vi "Generate View Regular Functions.vi"(8 "Error in":errorcluster, 9 "Table Name":string, 10 "Folder to Saved File":path, 11 "Connection in":refnum<class "Connection.lvclass">) -> (0 "Error out":errorcluster, 2 "SQL-LV File Paths":T1, 3 "Connection out":refnum<class "Connection.lvclass">)   [LabVIEW 2021]
uses:
  <vilib>/drjdpowell/SQLite Library/SQL Connection/Connection.lvclass
  SQL-LV View File Paths.ctl
  SQL-LV View Control Paths.ctl
  SQL-LV View VI Paths.ctl
  edt.lib/sqlite.lib/SQLite Field Info.ctl
  edt.lib/sqlite.lib/SQLite Data Type.ctl
  SQL-LV Table Control Paths.ctl
  Field Info to Cluster Item Info (Array).vi
  edt.lib/vie.lib/EDT VIE.lvlib
  edt.lib/sqlite.lib/EDT SQLite+.lvlib
  edt.lib/vi_script.lib/EDT VI Script.lvlib
panel:
  in  "Tab Control":enum32{"Main", "Misc"}(tab)
  out "itr":i32
  out "Previous State":string
  out "Current State":string
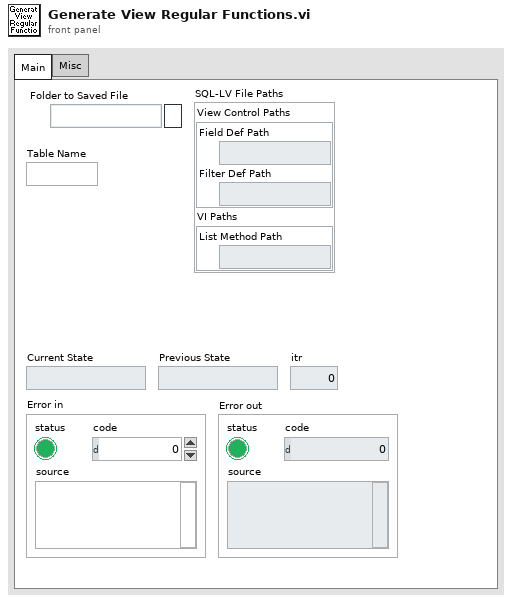
[diagram p1: front panel]
types:
  T1 = typedef "SQL-LV View File Paths.ctl" = cluster{"View Control Paths":T2, "VI Paths":T3}
  T2 = typedef "SQL-LV View Control Paths.ctl" = cluster{"Field Def Path":path, "Filter Def Path":path}
  T3 = typedef "SQL-LV View VI Paths.ctl" = cluster{"List Method Path":path}
  T4 = typedef "EDT SQLite+.lvlib/SQLite Field Info.ctl" = cluster{"cid":i32, "name":string, "type":T5, "notnull":bool, "dflt_value":variant, "pk":bool}
  T5 = typedef "EDT SQLite+.lvlib/SQLite Data Type.ctl" = enum16{"INT", "INTEGER", "TINYINT", "SMALLINT", "MEDIUMINT", "BIGINT", "UNSIGNED BIG INT", "INT2", "INT8", "CHARACTER", "VARCHAR", "VARYING CHARACTER", "NCHAR", "NATIVE CHARACTER", "NVARCHAR", "TEXT", "CLOB", "BLOB", "no datatype specified", "REAL", "DOUBLE", "DOUBLE PRECISION", "FLOAT", "NUMERIC", "DECIMAL", "BOOLEAN", "DATE", "DATETIME"}
  T6 = typedef "SQL-LV Table Control Paths.ctl" = cluster{"PK Def Path":path, "Data Def Path":path, "Field Def Path":path, "Filter Def Path":path}
  T7 = cluster{"Connection in":refnum<class "Connection.lvclass">, "Folder to Saved File":path, "Table Name":string, "SQL-LV File Paths":T1, "Fields Info":T4[]}
  T8 = typedef "EDT VI Script.lvlib/Cluster Item Info.ctl" = cluster{"Label.Text":string, "Type":T9, "Default Value":variant, "Description":string}
  T9 = typedef "NI_Data Type.lvlib/Data Type.ctl" = enum8{"Invalid Type", "Void", "I8", "I16", "I32", "I64", "U8", "U16", "U32", "U64", "Single Float", "Double Float", "Extended Float", "Single Complex", "Double Complex", "Extended Complex", "Enum U8", "Enum U16", "Enum U32", "Enum U64", "Single Float With Unit", "Double Float With Unit", "Extended Float With Unit", "Single Complex with Unit", "Double Complex with Unit", "Extended Complex with Unit", "Boolean", "String", "Path", "Picture", "Tag", "Array", "Cluster", "Variant", "LV Variant", "Waveform", "Timestamp", "Digital Waveform", "Digital Data", "ExpressData", "Refnum", "External Data", "VI", "Poly VI", "LabVIEW Class Instance", "Fixed Point", "Set Collection", "Map Collection"}
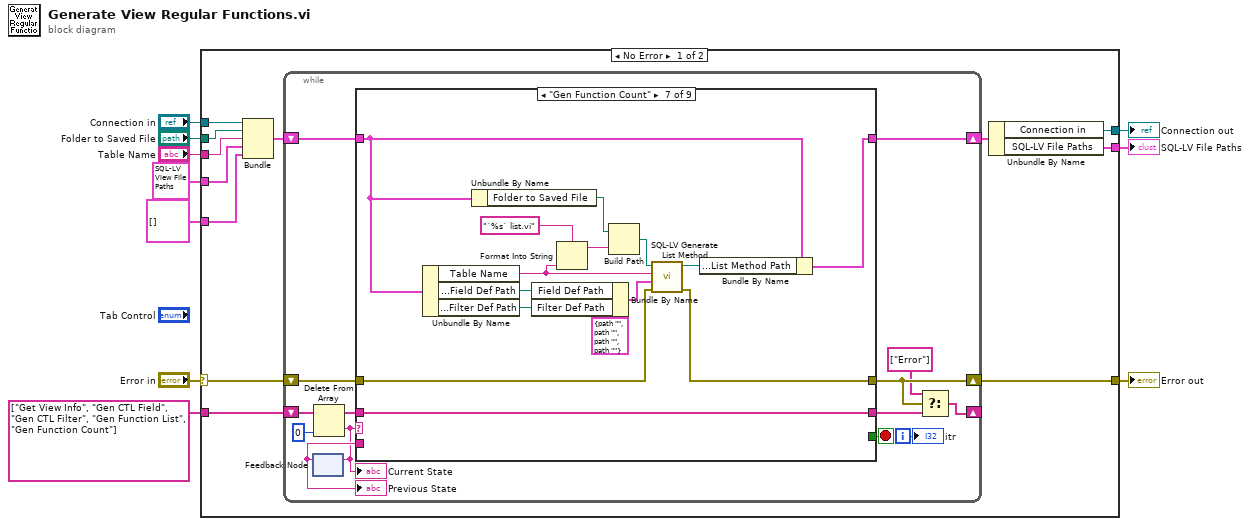
[diagram p0: block diagram]
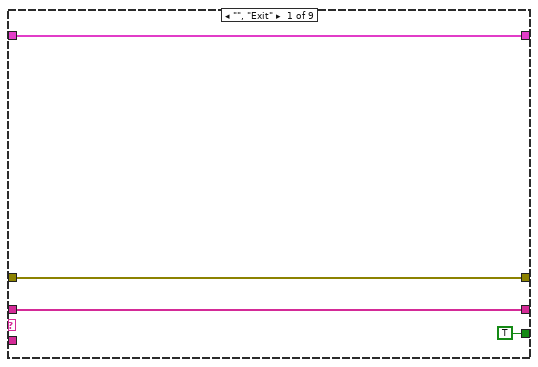
[diagram p2: hidden frame]
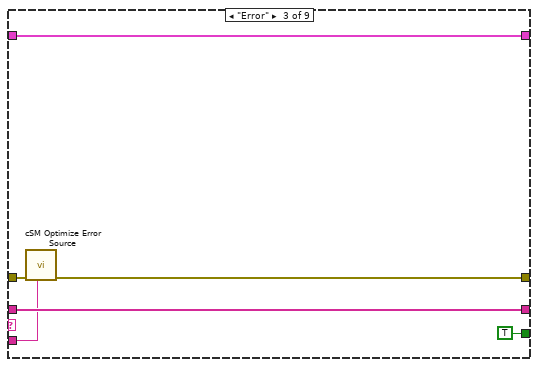
[diagram p4: hidden frame]
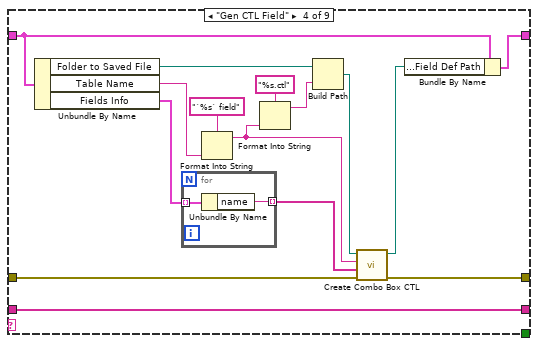
[diagram p5: hidden frame]
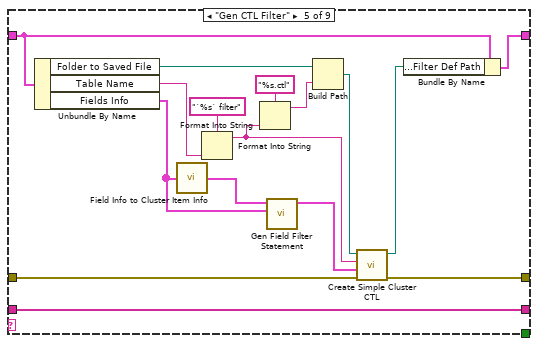
[diagram p6: hidden frame]
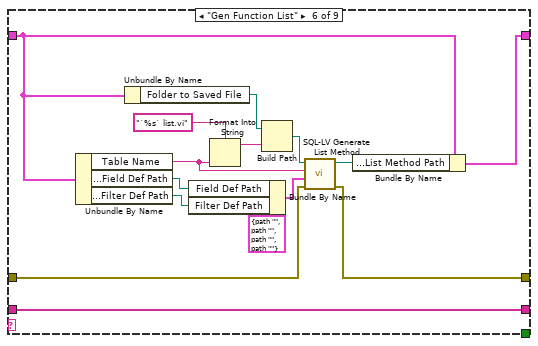
[diagram p7: hidden frame]
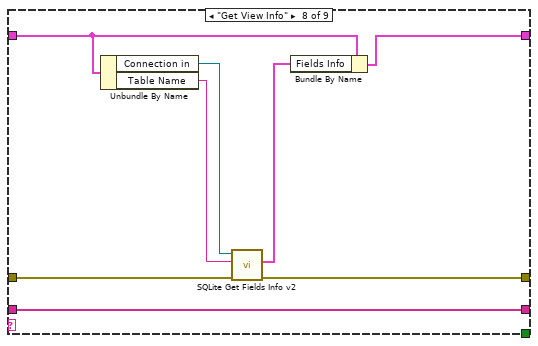
[diagram p8: hidden frame]
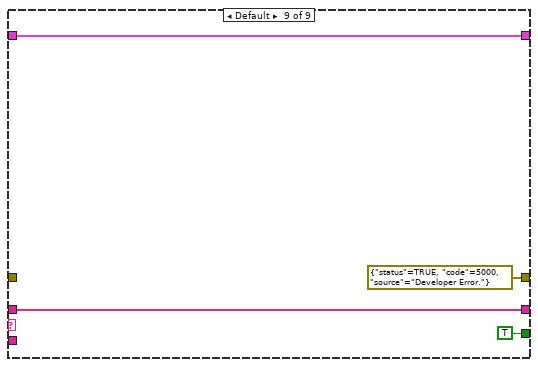
[diagram p9: hidden frame]
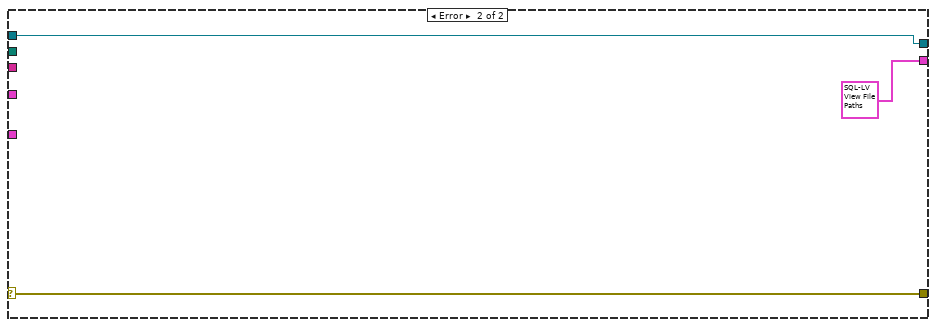
[diagram p10: hidden frame]
diagram:
  n1 = case shown="No Error" "Error in" {
    selector: "Error in" -> [w20 w127]
    tunnel: string[] ["Get View Info", "Gen CTL Field", "Gen CTL Filter", "Gen Function List", "Gen Function Count"] ("Initial States") -> [w22 _]
    tunnel: [w21 w127] -> w8
    tunnel: "Folder to Saved File" -> [w19 _]
    tunnel: "Table Name" -> [w18 _]
    tunnel: T1 {"View Control Paths"={"Field Def Path"=path "", "Filter Def Path"=path ""}, "VI Paths"={"List Method Path"=path ""}} ("SQL-LV File Paths") -> [w16 _]
    tunnel: [w14 T1 {"View Control Paths"={"Field Def Path"=path "", "Filter Def Path"=path ""}, "VI Paths"={"List Method Path"=path ""}} ("SQL-LV File Paths")] -> w4
    tunnel: T4[] [] ("Fields Info") -> [w13 _]
    tunnel: "Connection in" -> [w12 w126]
    tunnel: [w11 w126] -> w1
    frame No Error {
      n2 = Bundle("Connection in"=w12, "Folder to Saved File"=w19, "Table Name"=w18, "SQL-LV File Paths"=w16, "Fields Info"=w13) -> (w17:T7)  [unwired: 1 in]
      n3 = while {
        shift-right: [w30] -> _
        shift-left: w22 -> [w36]
        shift-right: [w29] -> w21
        shift-left: w20 -> [w33]
        shift-right: [w25] -> w15
        shift-left: w17 -> [w26]
        i -> [w34]
        stop <- w32 stop-if-true
        n4 = feedback #1() -> (w28:string)  [unwired: 1 in]
        "Previous State" <- w28
        n5 = Delete From Array(array=w36, index=0) -> (deleted portion=w27:string, array with subset deleted=w35:string[])  [unwired: 1 in]
        "Current State" <- w27
        n6 = feedback-in #1(w27) -> ()
        n7 = case shown="\"Gen Function Count\"" w27 {
          tunnel: [w40 w43 w49 w64 w82 w97 w112 w120 w122] -> w31
          tunnel: w35 -> [w40 w43 w49 w64 w82 w97 w112 w120 w122]
          tunnel: w33 -> [w39 w42 w47 w57 w76 w92 w107 w119 _]
          tunnel: [w39 w42 w46 w50 w67 w91 w106 w117 errorcluster {"status"=TRUE, "code"=5000, "source"="Developer Error."} ("error in")] -> w29
          tunnel: [TRUE _ TRUE _ _ _ _ _ TRUE] -> w32
          tunnel: w28 -> [_ _ w45 _ _ _ _ _ _]
          tunnel: w26 -> [w37 w41 w44 w63 w81 w90 w105 w116 w121]
          tunnel: [w37 w41 w44 w53 w72 w89 w104 w115 w121] -> w25
          frame "", "Exit" {
          }
          frame "<<KEEP>>" {
          }
          frame "Error" {
            n8 = call "cSM Optimize Error Source.vi"("Previous State"=w45, "Error in"=w47) -> ("Error out"=w46:errorcluster)  [unwired: 9 in]
          }
          frame "Gen CTL Field" {
            n9 = Unbundle By Name(w63) -> ("Folder to Saved File"=w55:path, "Table Name"=w60:string, "Fields Info"=w61:T4[])
            n10 = for {
              tunnel: w61 -> [w66] mode=indexing
              tunnel: [w65] -> w51 mode=indexing
              n11 = Unbundle By Name(w66) -> ("name"=w65:string)
            }
            n12 = Format Into String(format string="`%s` field", w60) -> (resulting string=w58:string)  [unwired: 2 in, 1 out]
            n13 = Format Into String(format string="%s.ctl", w58) -> (resulting string=w56:string)  [unwired: 2 in, 1 out]
            n14 = Build Path(base path=w55, name or relative path=w56) -> (appended path=w54:path)
            n15 = call "Create Combo Box CTL.vi"("error in (no error)"=w57, "Items"=w51, "Label Name"=w58, "Folder to Saved File"=w54) -> ("error out"=w50:errorcluster, "Path"=w52:path)  [unwired: 6 in]
            n16 = Bundle By Name(cluster=w63, "SQL-LV File Paths.View Control Paths.Field Def Path"=w52) -> (w53:T7)
          }
          frame "Gen CTL Filter" {
            n17 = Unbundle By Name(w81) -> ("Folder to Saved File"=w74:path, "Table Name"=w79:string, "Fields Info"=w68:T4[])
            n18 = call-poly "Field Info to Cluster Item Info.vi"("Fields Info"=w68) -> ("Cluster Items"=w70:T8[])
            n19 = Format Into String(format string="`%s` filter", w79) -> (resulting string=w77:string)  [unwired: 2 in, 1 out]
            n20 = Format Into String(format string="%s.ctl", w77) -> (resulting string=w75:string)  [unwired: 2 in, 1 out]
            n21 = call "Gen Field Filter Statement.vi"("Fields Info"=w68, "Cluster Items in"=w70) -> ("Cluster Items out"=w69:T8[])  [unwired: 9 in]
            n22 = Build Path(base path=w74, name or relative path=w75) -> (appended path=w73:path)
            n23 = call "Create Simple Cluster CTL.vi"("error in (no error)"=w76, "Cluster Item"=w69, "Label Name"=w77, "File Save Path"=w73) -> ("error out"=w67:errorcluster, "Path"=w71:path)  [unwired: 6 in]
            n24 = Bundle By Name(cluster=w81, "SQL-LV File Paths.View Control Paths.Filter Def Path"=w71) -> (w72:T7)
          }
          frame "Gen Function List" {
            n25 = Unbundle By Name(w90) -> ("Table Name"=w87:string, "SQL-LV File Paths.View Control Paths.Field Def Path"=w85:path, "SQL-LV File Paths.View Control Paths.Filter Def Path"=w84:path)
            n26 = Unbundle By Name(w90) -> ("Folder to Saved File"=w95:path)
            n27 = Bundle By Name(cluster=T6 {"PK Def Path"=path "", "Data Def Path"=path "", "Field Def Path"=path "", "Filter Def Path"=path ""} ("SQL-LV Control Paths"), "Field Def Path"=w85, "Filter Def Path"=w84) -> (w83:T6)
            n28 = Format Into String(format string="`%s` list.vi", w87) -> (resulting string=w94:string)  [unwired: 2 in, 1 out]
            n29 = Build Path(base path=w95, name or relative path=w94) -> (appended path=w93:path)
            n30 = call "SQL-LV Generate List Method.vi"("error in (no error)"=w92, "SQL-LV Control Paths"=w83, "Table Name"=w87, "Save as"=w93) -> ("error out"=w91:errorcluster, "Save as out"=w88:path)  [unwired: 6 in]
            n31 = Bundle By Name(cluster=w90, "SQL-LV File Paths.VI Paths.List Method Path"=w88) -> (w89:T7)
          }
          frame "Gen Function Count" {
            n32 = Unbundle By Name(w105) -> ("Table Name"=w102:string, "SQL-LV File Paths.View Control Paths.Field Def Path"=w100:path, "SQL-LV File Paths.View Control Paths.Filter Def Path"=w99:path)
            n33 = Unbundle By Name(w105) -> ("Folder to Saved File"=w110:path)
            n34 = Bundle By Name(cluster=T6 {"PK Def Path"=path "", "Data Def Path"=path "", "Field Def Path"=path "", "Filter Def Path"=path ""} ("SQL-LV Control Paths"), "Field Def Path"=w100, "Filter Def Path"=w99) -> (w98:T6)
            n35 = Format Into String(format string="`%s` list.vi", w102) -> (resulting string=w109:string)  [unwired: 2 in, 1 out]
            n36 = Build Path(base path=w110, name or relative path=w109) -> (appended path=w108:path)
            n37 = call "SQL-LV Generate List Method.vi"("error in (no error)"=w107, "SQL-LV Control Paths"=w98, "Table Name"=w102, "Save as"=w108) -> ("error out"=w106:errorcluster, "Save as out"=w103:path)  [unwired: 6 in]
            n38 = Bundle By Name(cluster=w105, "SQL-LV File Paths.VI Paths.List Method Path"=w103) -> (w104:T7)
          }
          frame "Get View Info" {
            n39 = Unbundle By Name(w116) -> ("Connection in"=w113:refnum<class "Connection.lvclass">, "Table Name"=w118:string)
            n40 = call "SQLite Get Fields Info v2.vi"("error in"=w119, "Table Name"=w118, "SQLite Connection"=w113) -> ("error out"=w117:errorcluster, "Fields Info"=w114:T4[])  [unwired: 6 in, 1 out]
            n41 = Bundle By Name(cluster=w116, "Fields Info"=w114) -> (w115:T7)
          }
          frame Default {
          }
        }
        n42 = Select(t=string[] ["Error"], s=w29, f=w31) -> (s? t:f=w30:string[])
        "itr" <- w34
      }
      n43 = Unbundle By Name(w15) -> ("Connection in"=w11:refnum<class "Connection.lvclass">, "SQL-LV File Paths"=w14:T1)
    }
    frame Error {
    }
  }
  "Error out" <- w8
  "Connection out" <- w1
  "SQL-LV File Paths" <- w4
